vi "Test State History.vi"() -> ()   [LabVIEW 2019]
uses:
  lvsrc/Framework/Instrument/Instrument.lvclass
panel:
  out "History":string
  in  "stop":bool
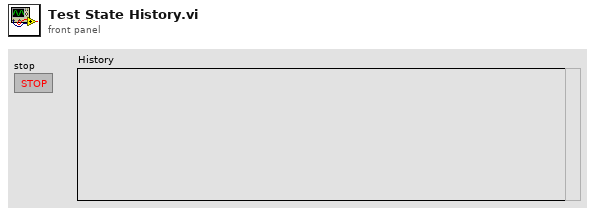
[diagram p1: front panel]
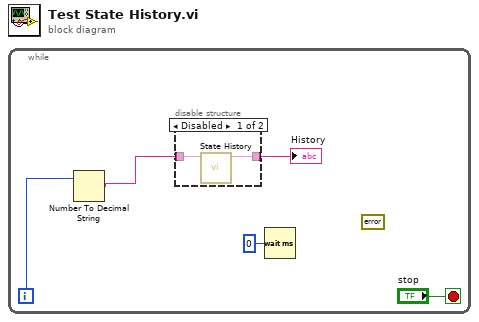
[diagram p0: block diagram]
diagram:
  n1 = while {
    i -> [w5]
    stop <- "stop" stop-if-true
    (unwired) errorcluster {"status"=FALSE, "code"=0, "source"=""} ("error constant")
    n2 = Number To Decimal String(number=w5) -> (decimal integer string=w4:string)  [unwired: 1 in]
    n3 = disable-structure shown="Disabled" {
      disable-tunnel: w4 -> [w7 _]
      disable-tunnel: [w6 _] -> w2
      frame Disabled {
        n4 = call "State History.vi"("Current State"=w7) -> ("History"=w6:string)  [unwired: 10 in]
      }
      frame Enabled {
      }
    }
    "History" <- w2
    n5 = Wait (ms)(milliseconds to wait=u32 0) -> ()  [unwired: 1 out]
  }
